vi "batting averade sub vi.vi"(6 "Other \nOuts":dbl, 9 "Base on \nError":dbl, 10 "strikeouts":dbl, 11 "hits":dbl) -> (3 "batting\naverage":dbl)   [LabVIEW 2018]
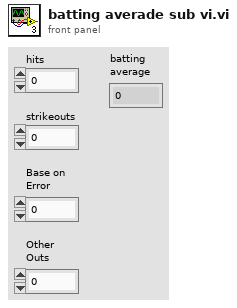
[diagram p1: front panel]
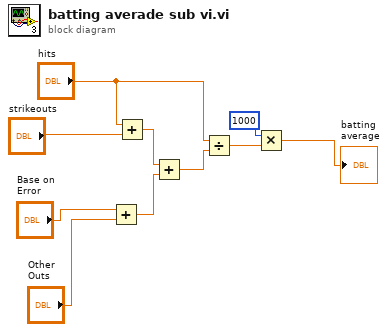
[diagram p0: block diagram]
diagram:
  n1 = Add(x="Base on \nError", y="Other \nOuts") -> (x+y=w5:dbl)
  n2 = Add(x="hits", y="strikeouts") -> (x+y=w4:dbl)
  n3 = Add(x=w4, y=w5) -> (x+y=w6:dbl)
  n4 = Divide(x="hits", y=w6) -> (x/y=w8:dbl)
  n5 = Multiply(x=1000, y=w8) -> (x*y=→"batting\naverage":dbl)
